vi "OpenStream.vi"(0 "data source rid":string, 1 "token":string) -> (7 "client handle out":T2, 8 "queue out":T1, 10 "error out":errorcluster)   [LabVIEW 2022 SP3]
uses:
  <vilib>/httpClient/LabVIEWHTTPClient.lvlib
  <vilib>/httpClient/ClientHandle.ctl
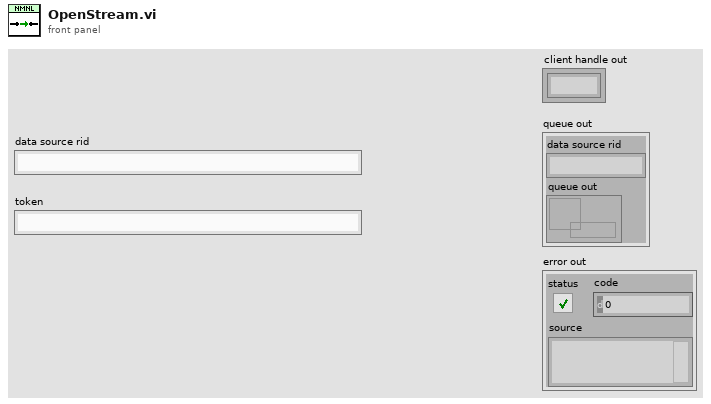
[diagram p1: front panel]
types:
  T1 = cluster{"data source rid":string, "queue out":refnum<queue>}
  T2 = typedef "LabVIEWHTTPClient.lvlib/ClientHandle.ctl" = refnum<k1>
  T3 = cluster{"channel":string, "time_seconds":i32, "time_nanos":i32, "value":dbl}
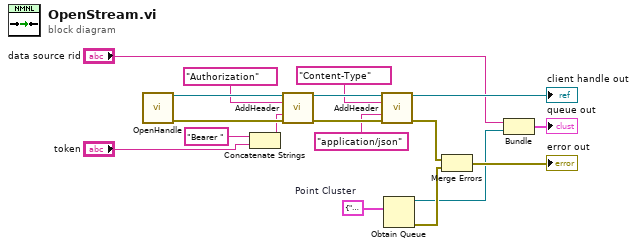
[diagram p0: block diagram]
diagram:
  w8 = T3 {"channel"="", "time_seconds"=0, "time_nanos"=0, "value"=0.0}  # Point Cluster
  n1 = call <vilib>:"OpenHandle.vi"() -> ("client handle out"=w13:T2, "error out"=w18:errorcluster)  [unwired: 14 in]
  n2 = Concatenate Strings("Bearer " ("value"), "token") -> (w15:string)
  n3 = call <vilib>:"AddHeader.vi"("client handle"=w13, "header"="Authorization", "value"=w15, "error in (no error)"=w18) -> ("client handle out"=w16:T2, "error out"=w17:errorcluster)  [unwired: 10 in]
  n4 = call <vilib>:"AddHeader.vi"("client handle"=w16, "header"="Content-Type", "value"="application/json", "error in (no error)"=w17) -> ("client handle out"=→"client handle out":T2, "error out"=w6:errorcluster)  [unwired: 10 in]
  n5 = Obtain Queue(element data type=w8) -> (queue out=w4:refnum<queue>, error out=w7:errorcluster)  [unwired: 4 in, 1 out]
  n6 = Merge Errors(w6, w7) -> (→"error out":errorcluster)
  n7 = Bundle("data source rid"="data source rid", "queue out"=w4) -> (→"queue out":T1)  [unwired: 1 in]
